vi "AG Spreadsheet Command.vi"(0 "error in":errorcluster, 1 "2D Data":string[][](array[string]), 2 "Data":string[](array[string]), 4 "Action (add)":T1=enum."Add") -> (7 "error out":errorcluster)   [LabVIEW 2010]
uses:
  Templates/AG Pages/Spreadsheet/Controls/Spreadsheet Commands.ctl
  Templates/AG Pages/Spreadsheet/Controls/Spreadsheet_Messege.ctl
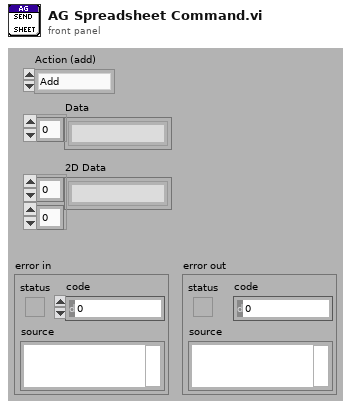
[diagram p1: front panel]
types:
  T1 = typedef "Spreadsheet Commands.ctl" = enum16{"Init", "Clear", "Add", "Mass Add", "Delete Row", "Format Colors", "Stop"}
  T2 = typedef "Spreadsheet_Messege.ctl" = cluster{"Action (add)":T1, "Data":string[], "2D Data":string[][]}
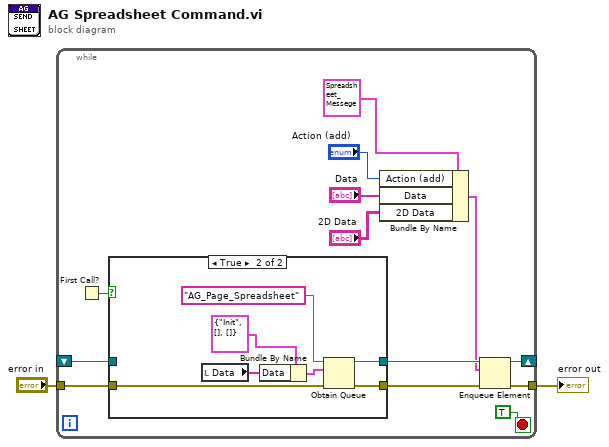
[diagram p0: block diagram]
diagram:
  n1 = while {
    shift-right: [w13] -> _
    shift-left: _ -> [w10]
    tunnel: "error in" -> [w9]
    tunnel: [w8] -> w1
    stop <- TRUE stop-if-true
    n2 = First Call?() -> (First Call?: T/F=w15:bool)
    n3 = case shown="True" w15 {
      tunnel: [w17 w23] -> w14
      tunnel: [w16 w22] -> w12
      tunnel: w10 -> [w17 _]
      tunnel: w9 -> [w16 w21]
      frame False {
      }
      frame True {
        n4 = local read "Data"() -> (w18:string[])
        n5 = Bundle By Name(cluster=T2 {"Action (add)"=enum."Init", "Data"=[], "2D Data"=[]} ("Cluster"), "Data"=w18) -> (w19:T2)
        n6 = Obtain Queue(name (unnamed)="AG_Page_Spreadsheet", element data type=w19, error in (no error)=w21) -> (queue out=w23:refnum<queue>, error out=w22:errorcluster)  [unwired: 2 in, 1 out]
      }
    }
    n7 = Bundle By Name(cluster=T2 {"Action (add)"=enum."Add", "Data"=["1", "2", "3", "4", "2345.56", "34.67"], "2D Data"=[]} ("Add"), "Action (add)"="Action (add)", "Data"="Data", "2D Data"="2D Data") -> (w3:T2)
    n8 = Enqueue Element(queue=w14, element=w3, error in (no error)=w12) -> (queue out=w13:refnum<queue>, error out=w8:errorcluster)  [unwired: 1 in, 1 out]
  }
  "error out" <- w1
